vi "Teleop.vi"(10 "Match Info":T1={"Autonomous Elapsed Seconds"=0.0, "TeleOp Elapsed Seconds"=0.0, "Disabled Elapsed Seconds"=0.0, "Visited Autonomous"=FALSE, "Visited TeleOp"=FALSE, "Visited Disabled"=FALSE, "Autonomous Settings"={"Autonomous Style"=enum."Independent", "VI Refnum"=refnum}}, 11 "Call Context":T2) -> ()   [LabVIEW 2014]
doc: "This VI is called for each TeleOp packet received from the DS where the robot is not disabled. It is often used to read from the joysticks and update I/O or to update setpoints for timed control loops. It should complete and return within 20 milliseconds or it may miss DS packets."
uses:
  <vilib>/Rock Robotics/WPI/DriverStation/WPI_DriverStationDerivedRobotMode.ctl
  <vilib>/Rock Robotics/WPI/DriverStation/WPI_DriverStationMatch Info.ctl
  <vilib>/Rock Robotics/WPI/Solenoid/WPI_SolenoidValue.ctl
  <vilib>/Rock Robotics/WPI/RobotDrive/WPI_RobotDriveGetSetRefNum.vi
  <vilib>/Rock Robotics/WPI/Joystick/WPI_JoystickGetSetRefNum.vi
  Robot Global Data.vi
  <vilib>/Rock Robotics/WPI/Solenoid/WPI_SolenoidSetEnum.vi
panel:
  out "Sample Slider 0":dbl(slide) scale=0.0..5.0
  out "Sample Boolean 1":bool
  out "Sample Boolean 0":bool
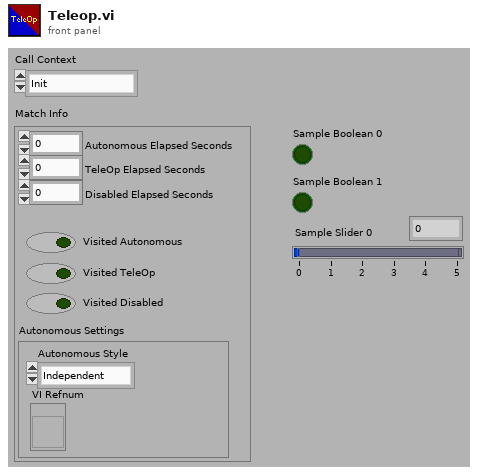
[diagram p1: front panel]
types:
  T1 = typedef "WPI_DriverStationMatch Info.ctl" = cluster{"Autonomous Elapsed Seconds":dbl, "TeleOp Elapsed Seconds":dbl, "Disabled Elapsed Seconds":dbl, "Visited Autonomous":bool, "Visited TeleOp":bool, "Visited Disabled":bool, "Autonomous Settings":cluster{"Autonomous Style":enum16{"Iterative", "Independent"}, "VI Refnum":refnum<vi>}}
  T2 = typedef "WPI_DriverStationDerivedRobotMode.ctl" = enum16{"Init", "Execute", "Stop"}
  T3 = typedef "WPI_SolenoidValue.ctl" = enum16{"Off", "On", "Forward", "Reverse"}
  T4 = typedef "WPI_RobotDriveDevRef.ctl" = cluster{"DevStatus":errorcluster, "Motors[]":T5[], "Square Inputs":bool, "Max Output":dbl}
  T5 = typedef "WPI_MotorControlDeviceRef.ctl" = cluster{"DeviceStatus":errorcluster, "Type":enum16{"PWM", "CAN"}, "PWM":cluster{"Digital Module":T6, "PWM Channel":T7, "DeadBand":T8}, "CAN":cluster{"Device Number":u8, "Control Mode":T9, "Semaphore":T10, "Max Vout":dbl}, "Invert":bool, "TransformRef":T11, "InvTransformRef":T11}
  T6 = typedef "FPGA_TypedefDigitalModule.ctl" = enum16{"Digital Module 1", "Digital Module 2"}
  T7 = typedef "FPGA_DIOPWMChannel.ctl" = enum8{"PWM 1", "PWM 2", "PWM 3", "PWM 4", "PWM 5", "PWM 6", "PWM 7", "PWM 8", "PWM 9", "PWM 10", "Invalid"}
  T8 = typedef "WPI_PWMDeadband.ctl" = cluster{"Name":string, "maxPositivePwm":i32, "minPositivePwm":i32, "centerPwm":i32, "maxNegativePwm":i32, "minNegativePwm":i32, "angularRange":u16}
  T9 = typedef "WPI_CANJaguar_ControlMode.ctl" = enum8{"Percent VBus", "Current", "Speed", "Position", "Voltage"}
  T10 = typedef "Semaphore RefNum" = refnum<k1>
  T11 = typedef "WPI_PWMTransform_ConPane.ctl" = refnum<vi>
  T12 = typedef "WPI_JoystickDevRef.ctl" = cluster{"Device":T13}
  T13 = typedef "WPI_JoystickDeviceEnum.ctl" = enum16{"USB 0", "USB 1", "USB 2", "USB 3", "USB 4", "USB 5"}
  T14 = typedef "WPI_SolenoidDevRef.ctl" = cluster{"DevStatus":errorcluster, "Solenoid Module":T15, "Forward Solenoid Channel":T16, "Reverse Solenoid Channel":T16}
  T15 = typedef "FPGA_TypedefSolenoidModule.ctl" = enum16{"Solenoid Module 1", "Solenoid Module 2"}
  T16 = typedef "WPI_SolenoidChannel.ctl" = enum8{"Solenoid 1", "Solenoid 2", "Solenoid 3", "Solenoid 4", "Solenoid 5", "Solenoid 6", "Solenoid 7", "Solenoid 8", "Invalid"}
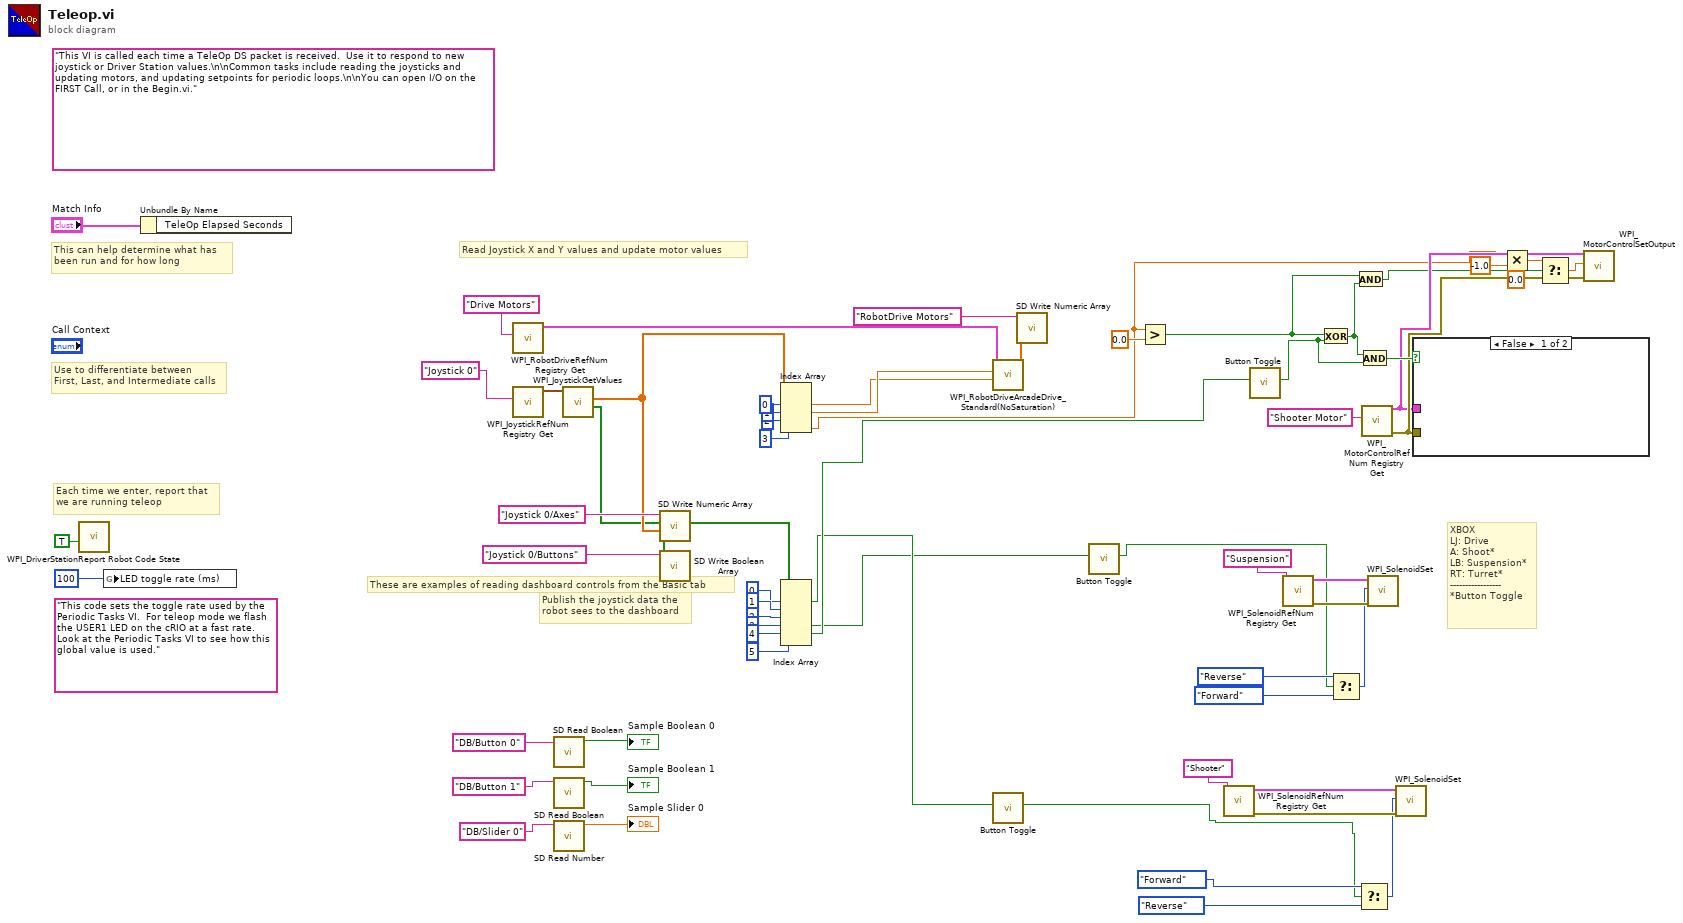
[diagram p0: block diagram]
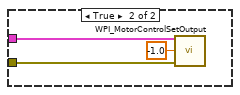
[diagram p2: hidden frame]
diagram:
  (unwired) "This code sets the toggle rate used by the Periodic Tasks VI.  For teleop mode we flash the USER1 LED on the cRIO at a fast rate.  Look at the Periodic Tasks VI to see how this global value is used."
  (unwired) "This VI is called each time a TeleOp DS packet is received.  Use it to respond to new joystick or Driver Station values.\n\nCommon tasks include reading the joysticks and updating motors, and updating setpoints for periodic loops.\n\nYou can open I/O on the FIRST Call, or in the Begin.vi."
  # "XBOX\nLJ: Drive\nA: Shoot*\nLB: Suspension*\nRT: Turret*\n-----------------\n*Button Toggle"
  # "These are examples of reading dashboard controls from the Basic tab"
  # "Publish the joystick data the\nrobot sees to the dashboard"
  # "Each time we enter, report that\nwe are running teleop"
  # "Use to differentiate between\nFirst, Last, and Intermediate calls"
  # "This can help determine what has\nbeen run and for how long"
  # "Read Joystick X and Y values and update motor values"
  n1 = call <vilib>:"WPI_DriverStationReport Robot Code State.vi"("TeleOp"=TRUE ("Autonomous")) -> ()  [unwired: 10 in, 1 out]
  n2 = global write "Robot Global Data.vi" "LED toggle rate (ms)"(u32 100 ("LED ms toggle rate")) -> ()
  n3 = Unbundle By Name("Match Info") -> ()  [unwired: 1 out]
  n4 = call <vilib>:"WPI_RobotDriveRefNum Registry Get.vi"("refnum name"="Drive Motors") -> ("RobotDriveDevRef"=w60:T4)  [unwired: 1 in, 9 out]
  n5 = call <vilib>:"WPI_JoystickRefNum Registry Get.vi"("refnum name"="Joystick 0") -> ("JoystickDevRef"=w58:T12)  [unwired: 1 in, 9 out]
  n6 = call <vilib>:"SD Read Boolean.vi"("Name"="DB/Button 0" ("refnum name")) -> ("Boolean"=→"Sample Boolean 0":bool)  [unwired: 8 in, 2 out]
  n7 = call <vilib>:"SD Read Boolean.vi"("Name"="DB/Button 1" ("refnum name")) -> ("Boolean"=→"Sample Boolean 1":bool)  [unwired: 8 in, 2 out]
  n8 = call <vilib>:"SD Read Number.vi"("Name"="DB/Slider 0" ("refnum name")) -> ("Numeric"=→"Sample Slider 0":dbl)  [unwired: 8 in, 2 out]
  n9 = call <vilib>:"WPI_JoystickGetValues.vi"("JoystickDevRef"=w58) -> ("Buttons"=w27:bool[], "Axes"=w28:dbl[])  [unwired: 6 in, 3 out]
  n10 = call <vilib>:"SD Write Numeric Array.vi"("Numeric Array"=w28, "Name"="Joystick 0/Axes") -> ()  [unwired: 8 in, 2 out]
  n11 = call <vilib>:"SD Write Boolean Array.vi"("Boolean Array"=w27, "Name"="Joystick 0/Buttons") -> ()  [unwired: 8 in, 2 out]
  n12 = Index Array(array=w28, index #1=0 ("index"), index #2=1 ("index"), index #3=2 ("index"), index #4=3 ("index")) -> (element #1=w29:dbl, element #2=w30:dbl, element #4=w6:dbl)  [unwired: 1 out]
  n13 = Index Array(array=w27, index #1=0 ("index"), index #2=1 ("index"), index #3=2 ("index"), index #4=3 ("index"), index #5=4 ("index"), index #6=5 ("index")) -> (element #1=w17:bool, element #4=w16:bool, element #5=w19:bool)  [unwired: 3 out]
  n14 = call <vilib>:"WPI_RobotDriveArcadeDrive_Standard(NoSaturation).vi"("Y axis value"=w29, "X axis value"=w30, "RobotDriveDevRef"=w60) -> ("Motor Values"=w53:dbl[])  [unwired: 1 in, 7 out]
  n15 = call "Button Toggle.vi"("Input"=w17) -> ("Output"=w18:bool)  [unwired: 10 in]
  n16 = call <vilib>:"SD Write Numeric Array.vi"("Numeric Array"=w53, "Name"="RobotDrive Motors") -> ()  [unwired: 8 in, 2 out]
  n17 = call "Button Toggle.vi"("Input"=w16) -> ("Output"=w15:bool)  [unwired: 10 in]
  n18 = Greater?(x=w6, y=0.0) -> (0:w12:bool)
  n19 = call <vilib>:"WPI_SolenoidRefNum Registry Get.vi"("refnum name"="Shooter") -> ("error out"=w44:errorcluster, "SolenoidDevRef"=w43:T14)  [unwired: 9 in]
  n20 = call "Button Toggle.vi"("Input"=w19) -> ("Output"=w9:bool)  [unwired: 10 in]
  n21 = call <vilib>:"WPI_SolenoidRefNum Registry Get.vi"("refnum name"="Suspension") -> ("error out"=w38:errorcluster, "SolenoidDevRef"=w37:T14)  [unwired: 9 in]
  n22 = Exclusive Or(1:w9, 2:w12) -> (0:w10:bool)
  n23 = Select(t=WPI_SolenoidValue."Reverse" ("Value"), s=w15, f=WPI_SolenoidValue."Forward") -> (s? t:f=w35:T3)
  n24 = And(x=w12, y=w10) -> (x .and. y?=w2:bool)
  n25 = Select(t=WPI_SolenoidValue."Forward" ("Value"), s=w18, f=WPI_SolenoidValue."Reverse") -> (s? t:f=w41:T3)
  n26 = And(x=w10, y=w9) -> (x .and. y?=w11:bool)
  n27 = call <vilib>:"WPI_MotorControlRefNum Registry Get.vi"("refnum name"="Shooter Motor") -> ("error out"=w8:errorcluster, "MotorControlDevRef"=w7:T5)  [unwired: 9 in]
  n28 = call-poly <vilib>:"WPI_SolenoidSet.vi"("error in (no error)"=w38, "Value"=w35, "SolenoidDevRef"=w37) -> ()  [unwired: 7 in, 2 out]
  n29 = call-poly <vilib>:"WPI_SolenoidSet.vi"("error in (no error)"=w44, "Value"=w41, "SolenoidDevRef"=w43) -> ()  [unwired: 7 in, 2 out]
  n30 = case shown="False" w11 {
    tunnel: w8 -> [_ w64]
    tunnel: w7 -> [_ w63]
    frame False {
    }
    frame True {
      n31 = call <vilib>:"WPI_MotorControlSetOutput.vi"("error in (no error)"=w64, "Output"=-1.0, "MotorControlDevRef"=w63) -> ()  [unwired: 6 in, 3 out]
    }
  }
  n32 = Multiply(x=w6, y=-1.0) -> (x*y=w4:dbl)
  n33 = Select(t=w4, s=w2, f=0.0) -> (s? t:f=w3:dbl)
  n34 = call <vilib>:"WPI_MotorControlSetOutput.vi"("error in (no error)"=w8, "Output"=w3, "MotorControlDevRef"=w7) -> ()  [unwired: 6 in, 3 out]
